vi "Execute.vi"(8 "error in (no error)":errorcluster, 11 "Node in":refnum<class "bt_WaitOn_Notifier.lvclass">) -> (0 "error out":errorcluster, 1 "Status":T1, 3 "Node out":refnum<class "bt_WaitOn_Notifier.lvclass">)   [LabVIEW 2021, in "BT.lvlib" / "bt_WaitOn_Notifier.lvclass"]
uses:
  bt_WaitOn_Notifier.lvclass
  C:/Users/Tim/Documents/GitHub/LV_Behaviour_Tree/Source/Support/Nodes/Leaves/Synch/Parent/WaitOn/bt_WaitOn_Synch.lvclass
  abs_Node/Status.ctl
  Parent/WaitOn/bt_WaitOn_Synch.lvclass/bt_WaitOn_Synch.ctl
  bt_WaitOn_Notifier.lvclass/bt_WaitOn_Notifier.ctl
  abs_Node/bt_Node.lvclass
  Parent/WaitOn/bt_WaitOn_Synch.lvclass
  With Values/WaitOn/bt_WaitOn_Synch_WithValues.lvclass
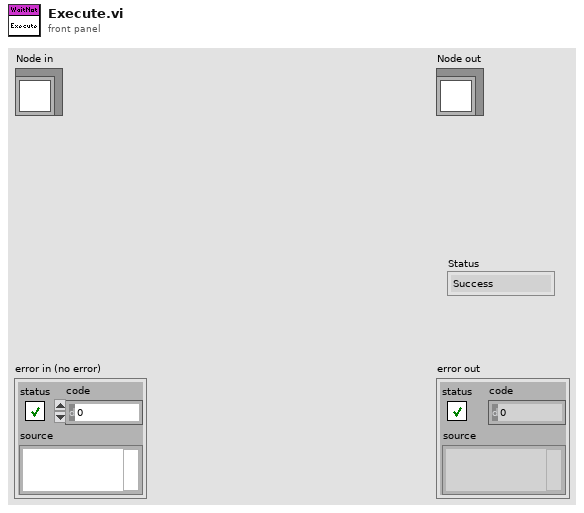
[diagram p1: front panel]
types:
  T1 = typedef "BT.lvlib/bt_Node.lvclass/Status.ctl" = enum16{"Success", "Failure", "Running"}
  T2 = typedef "NI_Data Type.lvlib/Data Type.ctl" = enum8{"Invalid Type", "Void", "I8", "I16", "I32", "I64", "U8", "U16", "U32", "U64", "Single Float", "Double Float", "Extended Float", "Single Complex", "Double Complex", "Extended Complex", "Enum U8", "Enum U16", "Enum U32", "Enum U64", "Single Float With Unit", "Double Float With Unit", "Extended Float With Unit", "Single Complex with Unit", "Double Complex with Unit", "Extended Complex with Unit", "Boolean", "String", "Path", "Picture", "Tag", "Array", "Cluster", "Variant", "LV Variant", "Waveform", "Timestamp", "Digital Waveform", "Digital Data", "ExpressData", "Refnum", "External Data", "VI", "Poly VI", "LabVIEW Class Instance", "Fixed Point", "Set Collection", "Map Collection"}
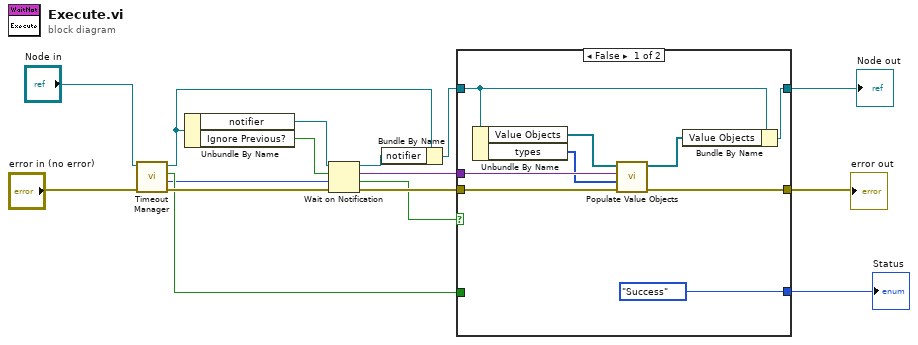
[diagram p0: block diagram]
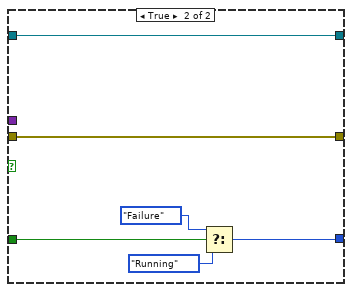
[diagram p2: hidden frame]
diagram:
  n1 = call "Timeout Manager.vi"("error in (no error)"="error in (no error)", "bt_WaitOn_Synch in"="Node in") -> ("error out"=w13:errorcluster, "Timeout"=w5:i32, "Timeout Now?"=w10:bool, "bt_WaitOn_Synch out"=w11:refnum<class "bt_WaitOn_Notifier.lvclass">)  [unwired: 5 in, 1 out]
  n2 = Unbundle By Name(w11) -> ("notifier"=w16:refnum<notifier>, "Ignore Previous?"=w1:bool)
  n3 = Wait on Notification(notifier=w16, ignore previous (F)=w1, timeout in ms (-1)=w5, error in (no error)=w13) -> (notifier out=w15:refnum<notifier>, notification=w2:variant, timed out?=w3:bool, error out=w4:errorcluster)
  n4 = Bundle By Name(cluster=w11, "notifier"=w15) -> (w7:refnum<class "bt_WaitOn_Notifier.lvclass">)
  n5 = case shown="False" w3 {
    tunnel: w4 -> [w24 w27]
    tunnel: w10 -> [_ w30]
    tunnel: [Status."Success" ("Status") w28] -> w9
    tunnel: [w23 w27] -> w8
    tunnel: w2 -> [w22 _]
    tunnel: w7 -> [w19 w26]
    tunnel: [w17 w26] -> w6
    frame False {
      n6 = Unbundle By Name(w19) -> ("Value Objects"=w21:refnum<class "Abs_Value.lvclass">[], "types"=w20:T2[])
      n7 = call "Populate Value Objects.vi"("error in (no error)"=w24, "LabVIEW types"=w20, "Variant"=w22, "Value Objects Type"=w21) -> ("error out"=w23:errorcluster, "Value Objects Out"=w18:refnum<class "Abs_Value.lvclass">[])  [unwired: 6 in]
      n8 = Bundle By Name(cluster=w19, "Value Objects"=w18) -> (w17:refnum<class "bt_WaitOn_Notifier.lvclass">)
    }
    frame True {
      n9 = Select(t=Status."Failure" ("Status"), s=w30, f=Status."Running") -> (s? t:f=w28:T1)
    }
  }
  "error out" <- w8
  "Node out" <- w6
  "Status" <- w9
